vi "Array_1.vi"() -> ()   [LabVIEW 2023]
panel:
  out "삭제된 배열":string[](array[string])
  out "부분이 삭제된 배열":string[](array[string])
  out "배열에 삽입":string[](array[string])
  out "부분 대체":string[](array[string])
  out "배열 인덱스":string
  out "크기":i32
  in  "Array":string[](array[string])
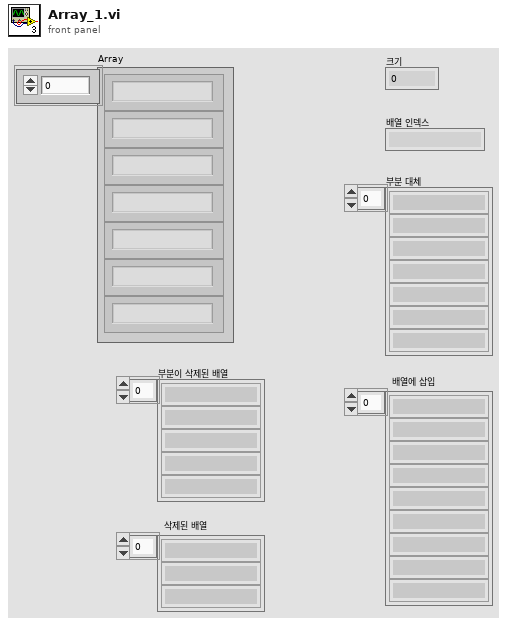
[diagram p1: front panel]
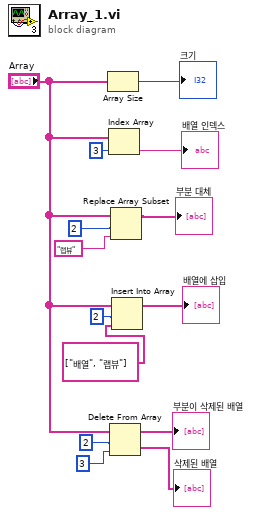
[diagram p0: block diagram]
diagram:
  n1 = Array Size(array="Array") -> (size(s)=→"크기":i32)
  n2 = Index Array(array="Array", index=3) -> (element=→"배열 인덱스":string)
  n3 = Delete From Array(array="Array", length=2, index=3) -> (deleted portion=→"삭제된 배열":string[], array with subset deleted=→"부분이 삭제된 배열":string[])
  n4 = Replace Array Subset(array="Array", new element="랩뷰" ("new element/subarray"), index=2) -> (→"부분 대체":string[])
  n5 = Insert Into Array(array="Array", index=2, new element=string[] ["배열", "랩뷰"]) -> (→"배열에 삽입":string[])
